vi "ExposeSend.vi"(0 "Expose":T1, 5 "Message":T2 {"Message Type" items=["Error"=1, "Warning"=2, "Create"=4, "Destroy"=8, "Invoke"=16, "Get"=32, "Set"=64, "Response"=128]}, 7 "Require Response":bool, 9 "HandlerID":string, 11 "error in (no error)":errorcluster) -> (4 "Expose out":T1, 6 "Response":T2 {"Message Type" items=["Error"=1, "Warning"=2, "Create"=4, "Destroy"=8, "Invoke"=16, "Get"=32, "Set"=64, "Response"=128]}, 15 "error out":errorcluster)   [LabVIEW 2017]
uses:
  ExposeMessage.ctl
  Events/ExposeMessageType.ctl
  Mapper/ExposeObjectMapNamepathData.ctl
  Mapper/ExposeMapperDataTypeEnum.ctl
  Mapper/ExposeObjectMapContainerTypeEnum.ctl
  ExposeInfo.ctl
  C:/Code/CMCryoSysCode/Expose/COM/CSCom/CSCom/bin/Release/CSCom.dll
  COM/CSCom/CSCom/bin/Release/CSCom.dll
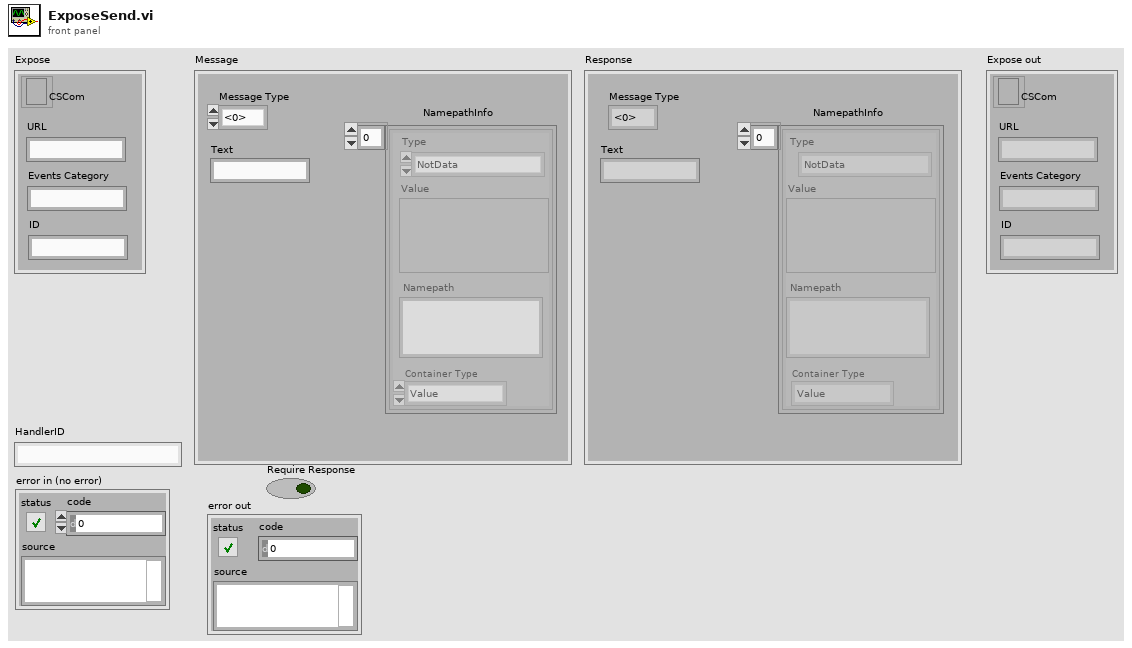
[diagram p1: front panel]
types:
  T1 = typedef "ExposeInfo.ctl" = cluster{"CSCom":refnum<k24>, "URL":string, "Events Category":string, "ID":string}
  T2 = typedef "ExposeMessage.ctl" = cluster{"Message Type":T3, "Text":string, "NamepathInfo":T4[]}
  T3 = typedef "ExposeMessageType.ctl" = i32
  T4 = typedef "ExposeObjectMapNamepathData.ctl" = cluster{"Type":T5, "Value":variant, "Namepath":string, "Container Type":T6}
  T5 = typedef "ExposeMapperDataTypeEnum.ctl" = enum16{"NotData", "int8", "byte", "int16", "uint16", "int32", "uint32", "int64", "uint64", "Single", "Double", "String", "Boolean", "Container"}
  T6 = typedef "ExposeObjectMapContainerTypeEnum.ctl" = enum16{"Value", "Array", "Waveform", "NetContainer"}
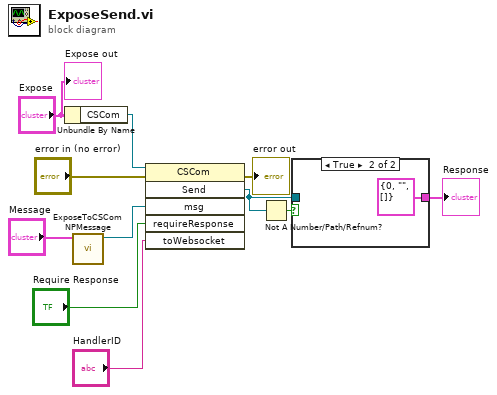
[diagram p0: block diagram]
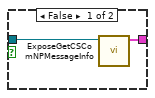
[diagram p2: hidden frame]
diagram:
  n1 = Unbundle By Name("Expose") -> ("CSCom"=w10:refnum<k24>)
  n2 = call "ExposeToCSComNPMessage.vi"("Message"="Message") -> (".NET Refnum out"=w3:refnum<k24>)  [unwired: 10 in]
  n3 = invoke class="CSCom" method="Send"(reference=w10, error in="error in (no error)", "msg"=w3, "requireResponse"="Require Response", "toWebsocket"="HandlerID") -> (error out=→"error out":errorcluster, "Send"=w2:refnum<k24>)  [unwired: 1 in, 4 out]
  n4 = Not A Number/Path/Refnum?(number/path/refnum=w2) -> (NaN/Path/Refnum?=w1:bool)
  n5 = case shown="True" w1 {
    tunnel: [w13 T2 {"Message Type"=0, "Text"="", "NamepathInfo"=[]} ("MessageInfo")] -> w6
    tunnel: w2 -> [w12 _]
    frame False {
      n6 = call "ExposeGetCSComNPMessageInfo.vi"("NPMessage"=w12) -> ("MessageInfo"=w13:T2)  [unwired: 10 in]
    }
    frame True {
    }
  }
  "Response" <- w6
  "Expose out" <- "Expose"
